vi "Speed conversion.vi"(11 "Filtered data":i32) -> (3 "Numeric":sgl)   [LabVIEW 2016]
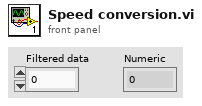
[diagram p1: front panel]
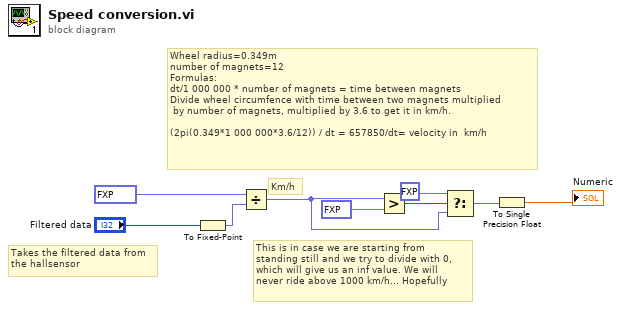
[diagram p0: block diagram]
diagram:
  # "Takes the filtered data from\nthe hallsensor"
  # "Wheel radius=0.349m\nnumber of magnets=12\nFormulas:\ndt/1 000 000 * number of magnets = time between magnets\nDivide wheel circumfence with time between two magnets multiplied\n by number of magnets, multiplied by 3.6 to get it in km/h.\n\n(2pi(0.349*1 000 000*3.6/12)) / dt = 657850/dt= velocity in  km/h"
  # "This is in case we are starting from\nstanding still and we try to divide with 0, \nwhich will give us an inf value. We will \nnever ride above 1000 km/h... Hopefully"
  # "Km/h"
  n1 = To Fixed-Point(number="Filtered data") -> (fixed-point=w5:fxp<+/-,32,32>)  [unwired: 1 in]
  n2 = Divide(x=fxp<+,19,20> 657850.0, y=w5) -> (x/y=w4:fxp<+/-,52,21>)
  n3 = Greater?(x=w4, y=fxp<+,7,10> 1000.0) -> (0:w2:bool)
  n4 = Select(t=fxp<+,1,1> 0.0, s=w2, f=w4) -> (s? t:f=w7:fxp<+/-,52,21>)
  n5 = To Single Precision Float(number=w7) -> (single precision float=→"Numeric":sgl)
